vi "FGC_Query.vi"(0 "System no.":i32=1 min=1 max=4 step=1, 2 "Routine name":string[](array[string]), 4 "Query all?":bool, 5 "error in":errorcluster) -> (14 "Scan axis center":dbl[](array[numeric]) format="%.6f", 15 "Step axis center":dbl[](array[numeric]) format="%.6f", 16 "Queried routine name out":string[](array[string]), 19 "error out":errorcluster)   [LabVIEW 2020]
doc: "Query fast alignment gradient search dither center values.\n\nC-887, E-712:"
panel:
  # "Query Fast Gradient scan dither Center"
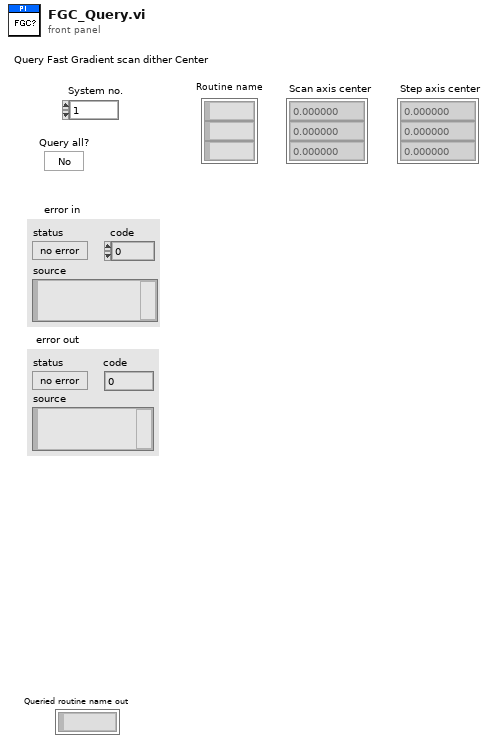
[diagram p1: front panel]
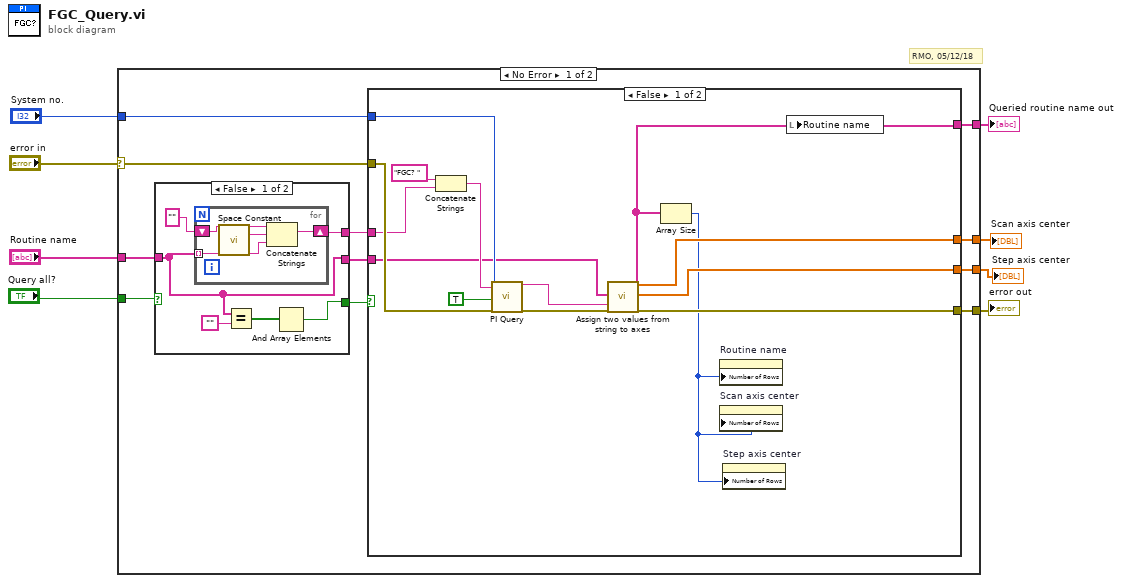
[diagram p0: block diagram]
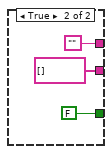
[diagram p2: hidden frame]
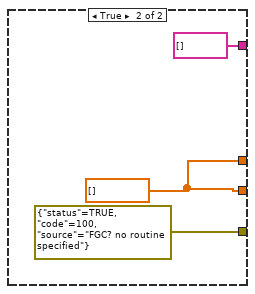
[diagram p3: hidden frame]
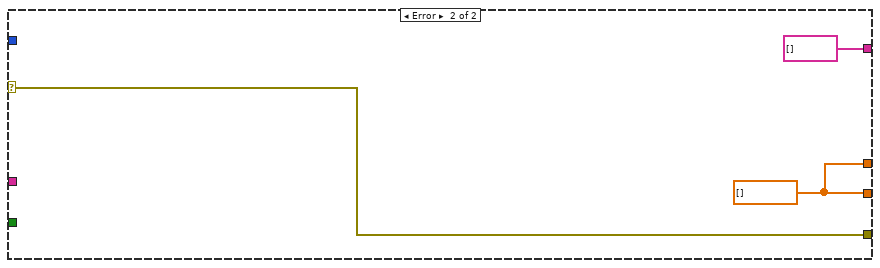
[diagram p4: hidden frame]
diagram:
  # "RMO, 05/12/18"
  n1 = case shown="No Error" "error in" {
    selector: "error in" -> [w9 w50]
    tunnel: "Routine name" -> [w19 _]
    tunnel: "System no." -> [w11 _]
    tunnel: [w17 w50] -> w6
    tunnel: [w15 w51] -> w5
    tunnel: "Query all?" -> [w14 _]
    tunnel: [w13 string[] [] ("Queried axes out")] -> w4
    tunnel: [w12 w51] -> w2
    frame No Error {
      n2 = case shown="False" w14 {
        tunnel: w19 -> [w21 _]
        tunnel: [w21 string[] [] ("Designator to query")] -> w18
        tunnel: [w20 FALSE] -> w16
        tunnel: [w22 "" ("Command substring")] -> w10
        frame False {
          n3 = for {
            shift-right: [w26] -> w22
            shift-left: "" -> [w29]
            tunnel: w21 -> [w27] mode=indexing
            n4 = call "Space Constant.vi"() -> ("String"=w28:string)
            n5 = Concatenate Strings(w29, w28, w27) -> (w26:string)
          }
          n6 = Equal?(x=w21, y="" ("x")) -> (x = y?=w24:bool[])
          n7 = And Array Elements(Boolean array=w24) -> (logical AND=w20:bool)
        }
        frame True {
        }
      }
      n8 = case shown="False" w16 {
        tunnel: w9 -> [w42 _]
        tunnel: w18 -> [w36 _]
        tunnel: w11 -> [w40 _]
        tunnel: [w39 errorcluster {"status"=TRUE, "code"=100, "source"="FGC? no routine specified"} ("error out")] -> w17
        tunnel: [w43 w47] -> w15
        tunnel: [w41 string[] [] ("Queried axes out")] -> w13
        tunnel: [w38 w47] -> w12
        tunnel: w10 -> [w35 _]
        frame False {
          n9 = Concatenate Strings("FGC? ", w35) -> (w44:string)
          n10 = call "PI Query.vi"("System no."=w40, "String to send"=w44, "Attach termination char.?"=TRUE ("Attach Linefeed?"), "error in"=w42) -> ("String read"=w34:string, "error out"=w33:errorcluster)  [unwired: 3 in, 11 out]
          n11 = call "Assign two values from string to axes.vi"("Queried axes"=w36, "Input String"=w34, "error in"=w33) -> ("Values 1"=w43:dbl[], "Values 2"=w38:dbl[], "Queried axes out"=w41:string[], "error out"=w39:errorcluster)  [unwired: 2 in, 11 out]
          n12 = Array Size(array=w41) -> (size(s)=w37:i32)
          n13 = property on="Routine name" class="Arr (strict)"("Number of Rows"=w37) -> ()  [unwired: 2 in, 2 out]
          n14 = property on="Scan axis center" class="Arr (strict)"("Number of Rows"=w37) -> ()  [unwired: 2 in, 2 out]
          n15 = property on="Step axis center" class="Arr (strict)"("Number of Rows"=w37) -> ()  [unwired: 2 in, 2 out]
          n16 = local write "Routine name"(w41) -> ()
        }
        frame True {
          w47 = dbl[] [] ("Parameter values")
        }
      }
    }
    frame Error {
      w51 = dbl[] [] ("Parameter values")
    }
  }
  "error out" <- w6
  "Scan axis center" <- w5
  "Queried routine name out" <- w4
  "Step axis center" <- w2
